vi "Load Complex Array From File.vi"(11 "file path (dialog if empty)":path) -> (3 "Array":cdb[](array[numeric]))   [LabVIEW 2011]
uses:
  <vilib>/Utility/file.llb/Read From Spreadsheet File (DBL).vi
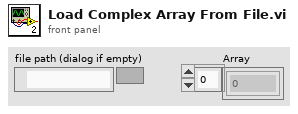
[diagram p1: front panel]
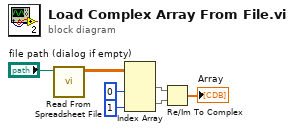
[diagram p0: block diagram]
diagram:
  n1 = call-poly <vilib>:"Read From Spreadsheet File.vi"("file path (dialog if empty)"="file path (dialog if empty)") -> ("all rows"=w2:dbl[][])  [unwired: 6 in, 4 out]
  n2 = Index Array(array=w2, index (col) #1=0 ("disabled index (col)"), index (col) #2=1 ("index (col)")) -> (element #1=w5:dbl[], element #2=w6:dbl[])  [unwired: 2 in]
  n3 = Re/Im To Complex(1:w6, 2:w5) -> (0:→"Array":cdb[])
